vi "corner_for_rectangle.vi"(9 "Y":dbl[](array[numeric]), 10 "X":dbl[](array[numeric]), 11 "Y Resolution":i32) -> (0 "area":dbl, 3 "corner":dbl[][](array[numeric]), 4 "length ratio":dbl)   [LabVIEW 2017]
panel:
  out "side distines":dbl[](array[numeric])
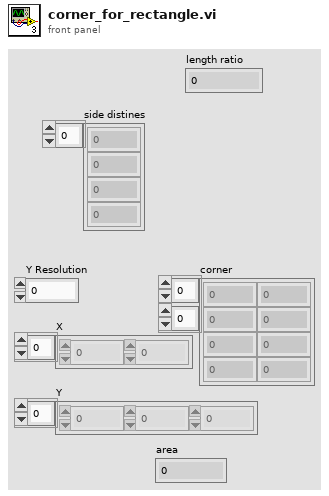
[diagram p1: front panel]
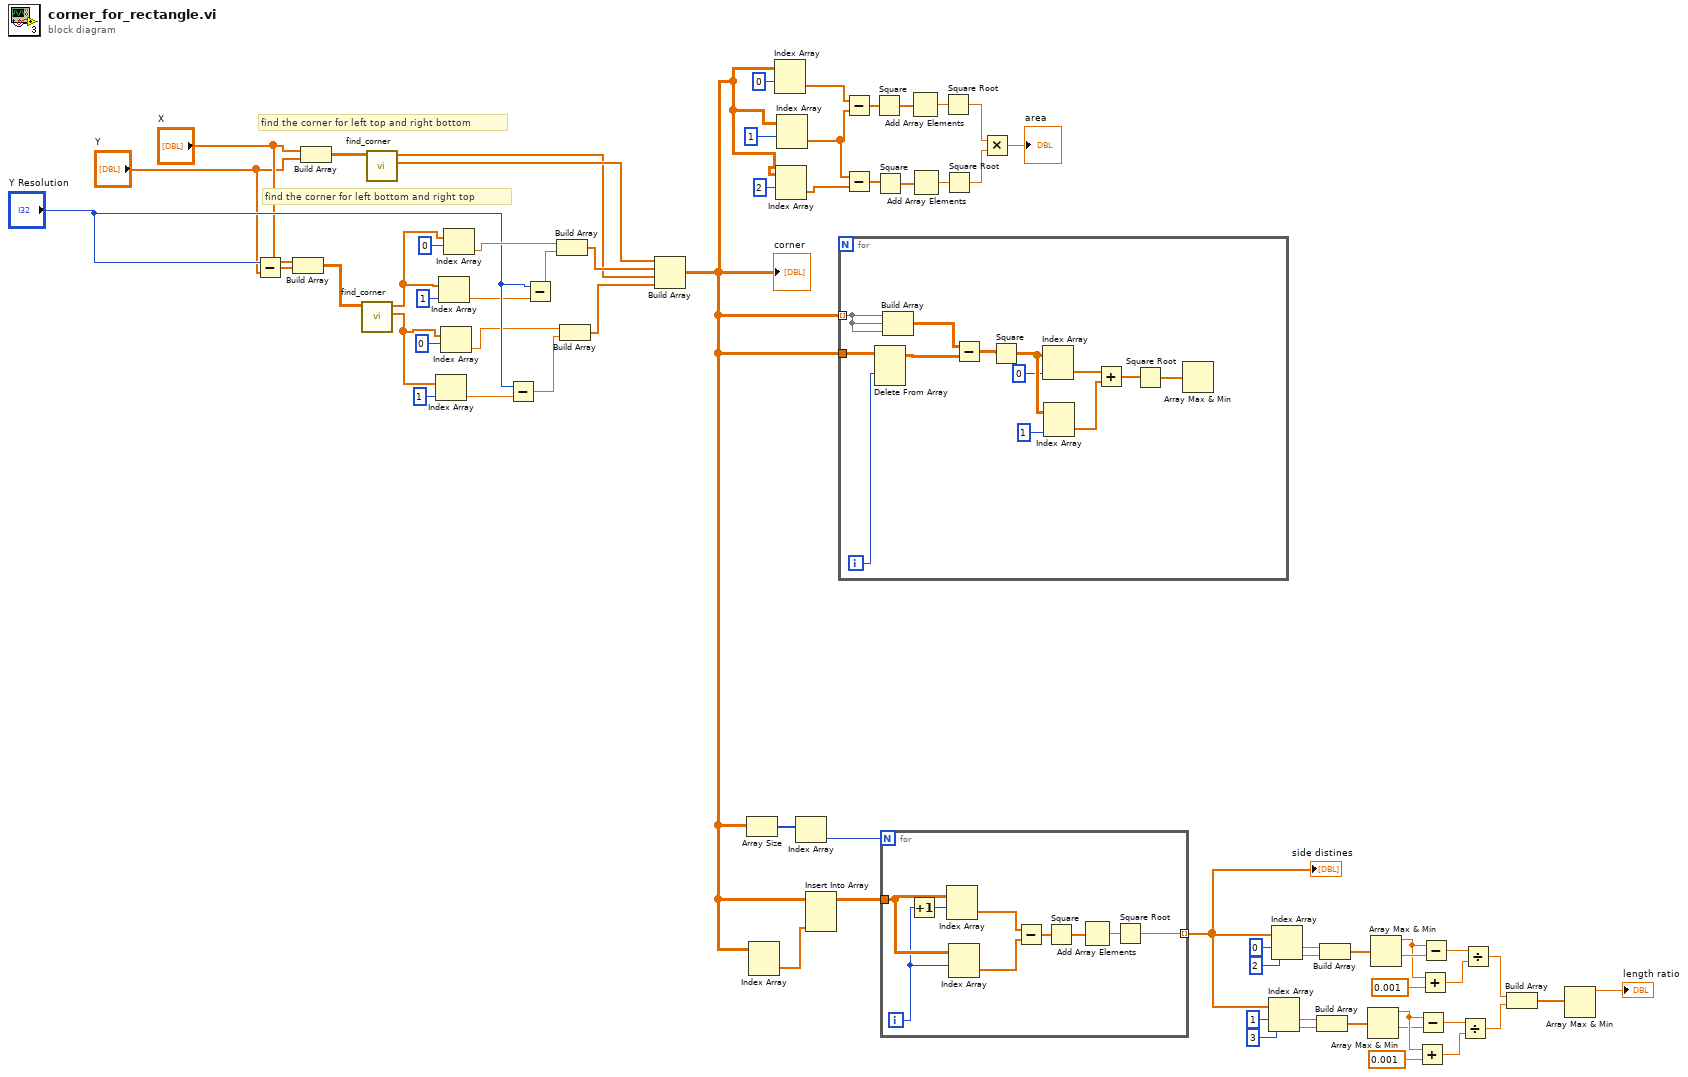
[diagram p0: block diagram]
diagram:
  # "find the corner for left bottom and right top"
  # "find the corner for left top and right bottom"
  n1 = Subtract(x="Y Resolution", y="Y") -> (x-y=w51:dbl[])
  n2 = Build Array("X", w51) -> (w52:dbl[][])
  n3 = Build Array("X", "Y") -> (w48:dbl[][])
  n4 = call "find_corner.vi"("XY in"=w52) -> ("left top"=w60:dbl[], "right bottom"=w61:dbl[])  [unwired: 9 in]
  n5 = call "find_corner.vi"("XY in"=w48) -> ("left top"=w66:dbl[], "right bottom"=w47:dbl[])  [unwired: 9 in]
  n6 = Index Array "Index Array"(array=w60, index=1) -> (element=w54:dbl)
  n7 = Index Array "Index Array"(array=w61, index=1) -> (element=w62:dbl)
  n8 = Index Array "Index Array"(array=w60, index=0) -> (element=w56:dbl)
  n9 = Index Array "Index Array"(array=w61, index=0) -> (element=w65:dbl)
  n10 = Subtract(x="Y Resolution", y=w54) -> (x-y=w57:dbl)
  n11 = Subtract(x="Y Resolution", y=w62) -> (x-y=w64:dbl)
  n12 = Build Array(w65, w64) -> (w67:dbl[])
  n13 = Build Array(w56, w57) -> (w46:dbl[])
  n14 = Build Array(w66, w67, w47, w46) -> (w26:dbl[][])
  "corner" <- w26
  n15 = Array Size(array=w26) -> (size(s)=w28:i32[])
  n16 = Index Array "Index Array"(array=w26) -> (element=w30:dbl[])  [unwired: 2 in]
  n17 = Index Array(array=w26, index (row)=0) -> (element=w43:dbl[])  [unwired: 1 in]
  n18 = Index Array(array=w26, index (row)=2) -> (element=w40:dbl[])  [unwired: 1 in]
  n19 = Index Array(array=w26, index (row)=1) -> (element=w41:dbl[])  [unwired: 1 in]
  n20 = Index Array "Index Array"(array=w28) -> (element=w27:i32)  [unwired: 1 in]
  n21 = Insert Into Array "Insert Into Array"(array=w26, new element=w30) -> (w29:dbl[][])  [unwired: 2 in]
  n22 = for {
    tunnel: w26 -> [w80] mode=indexing
    tunnel: w26 -> [w71]
    i -> [w68]
    n23 = Delete From Array(array=w71, index (row)=w68) -> (array with subset deleted=w69:dbl[][])  [unwired: 2 in, 1 out]
    n24 = Build Array(w80, w80, w80) -> (w70:dbl[][])
    n25 = Subtract(x=w70, y=w69) -> (x-y=w79:dbl[][])
    n26 = Square(x=w79) -> (x^2=w78:dbl[][])
    n27 = Index Array "Index Array"(array=w78, index (col)=0 ("index (row)")) -> (element=w75:dbl[])  [unwired: 1 in]
    n28 = Index Array(array=w78, index (col)=1 ("index (row)")) -> (element=w74:dbl[])  [unwired: 1 in]
    n29 = Add(x=w75, y=w74) -> (x+y=w73:dbl[])
    n30 = Square Root(x=w73) -> (sqrt(x)=w72:dbl[])
    n31 = Array Max & Min(array=w72) -> ()  [unwired: 4 out]
  }
  n32 = Subtract(x=w43, y=w41) -> (x-y=w39:dbl[])
  n33 = Subtract(x=w41, y=w40) -> (x-y=w34:dbl[])
  n34 = Square(x=w39) -> (x^2=w38:dbl[])
  n35 = Square(x=w34) -> (x^2=w35:dbl[])
  n36 = for {
    N: w27 -> [_]
    tunnel: w29 -> [w85]
    tunnel: [w81] -> w5 mode=indexing
    i -> [w84]
    n37 = Increment(x=w84) -> (x+1=w83:i32)
    n38 = Index Array "Index Array"(array=w85, index (row)=w83) -> (element=w89:dbl[])  [unwired: 1 in]
    n39 = Index Array(array=w85, index (row)=w84) -> (element=w82:dbl[])  [unwired: 1 in]
    n40 = Subtract(x=w89, y=w82) -> (x-y=w88:dbl[])
    n41 = Square(x=w88) -> (x^2=w87:dbl[])
    n42 = Add Array Elements(numeric array=w87) -> (sum=w86:dbl)
    n43 = Square Root(x=w86) -> (sqrt(x)=w81:dbl)
  }
  "side distines" <- w5
  n44 = Add Array Elements(numeric array=w38) -> (sum=w37:dbl)
  n45 = Add Array Elements(numeric array=w35) -> (sum=w36:dbl)
  n46 = Square Root(x=w37) -> (sqrt(x)=w33:dbl)
  n47 = Square Root(x=w36) -> (sqrt(x)=w32:dbl)
  n48 = Multiply(x=w33, y=w32) -> (x*y=→"area":dbl)
  n49 = Index Array(array=w5, index #1=1 ("index"), index #2=3 ("index")) -> (element #1=w8:dbl, element #2=w9:dbl)
  n50 = Index Array(array=w5, index #1=0 ("index"), index #2=2 ("index")) -> (element #1=w23:dbl, element #2=w22:dbl)
  n51 = Build Array(w8, w9) -> (w10:dbl[])
  n52 = Build Array(w23, w22) -> (w21:dbl[])
  n53 = Array Max & Min(array=w10) -> (max value=w14:dbl, min value=w12:dbl)  [unwired: 2 out]
  n54 = Array Max & Min(array=w21) -> (max value=w17:dbl, min value=w19:dbl)  [unwired: 2 out]
  n55 = Add(x=w14, y=0.001) -> (x+y=w15:dbl)
  n56 = Subtract(x=w14, y=w12) -> (x-y=w13:dbl)
  n57 = Add(x=w17, y=0.001) -> (x+y=w16:dbl)
  n58 = Subtract(x=w17, y=w19) -> (x-y=w18:dbl)
  n59 = Divide(x=w13, y=w15) -> (x/y=w3:dbl)
  n60 = Divide(x=w18, y=w16) -> (x/y=w4:dbl)
  n61 = Build Array(w4, w3) -> (w2:dbl[])
  n62 = Array Max & Min(array=w2) -> (max value=→"length ratio":dbl)  [unwired: 3 out]
